vi "modbus slave new.vi"() -> ()   [LabVIEW 2016]
uses:
  <vilib>/NI/Modbus Library/Network Protocol/Network Slave/daemon status.ctl
  <vilib>/NI/Modbus Library/Network Protocol/Network Slave/TCP/Connection.ctl
  <vilib>/NI/Modbus Library/API/Wrapper/Create TCP Slave.vi
  <vilib>/NI/Modbus Library/API/slave/Modbus Slave.lvclass
  <vilib>/NI/Modbus Library/API/Wrapper/API Main.lvlib
  <vilib>/ptbypt/NI_PtbyPt.lvlib
  <vilib>/Utility/config.llb/NI_LVConfig.lvlib
  <vilib>/NI/Modbus Library/Network Protocol/Network Slave/Network Slave.lvclass
  <vilib>/NI/Modbus Library/Network Protocol/Network Slave/TCP/TCP Slave.lvclass
panel:
  out "TCP Connection List":T1[](array[typedef])
  out "TCP Connection Count":u32
  out "Daemon Status":T2
  out "Daemon Error":errorcluster
  out "读取register values 2":u16[](array[numeric])
  out "status":bool
  in  "写入registers to write":u16[](array[numeric])
  out "读取register values":u16[](array[numeric])
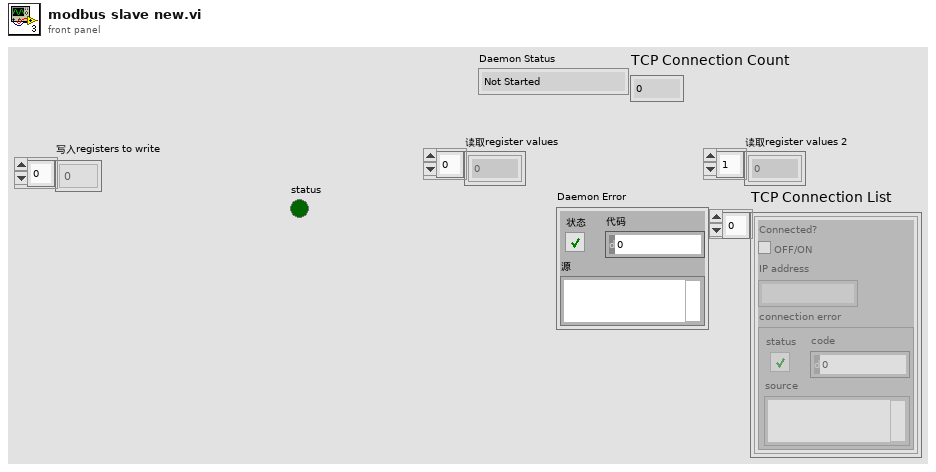
[diagram p1: front panel]
types:
  T1 = typedef "TCP Slave.lvclass/Connection.ctl" = cluster{"Connected?":bool, "IP address":string, "connection error":errorcluster}
  T2 = typedef "Network Slave.lvclass/daemon status.ctl" = enum16{"Not Started", "Running", "Error", "Stopped"}
  T3 = enum16{"启动整机", "停止整机", "标样核查", "加标回收", "平行样测试", "零点核查", "跨度核查", "校零", "校标"}
  T4 = cluster{"status":bool, "代码":u16, "source":string}
  T5 = cluster{"COD浓度（mg/L)":dbl, "水样启动时间":timestamp, "加标回收启动时间":timestamp, "CODMn工作状态":enum16{"空闲", "水样测试", "标样核查", "零点核查", "跨度核查", "空白测试", "平行样测试", "加标回收", "空白校准", "标样校准", "初始化（清洗）"}, "多列列表框":i32}
  T6 = cluster{"系统时间":timestamp, "工作状态":enum16{"空闲", "水样测试", "标样核查", "零点核查", "跨度核查", "空白测试", "平行样测试", "加标回收", "空白校准", "标样校准", "初始化（清洗）"}, "测量模式":enum16{"待机", "连续模式", "周期模式", "定点模式", "受控模式", "手动模式"}, "告警代码":u16, "故障代码":u16, "日志代码":u16, "软件版本":u16, "F0":sgl, "F1":sgl, "F2":sgl, "F3":sgl, "T":sgl, "H":sgl, "id":u16, "flowid":u16, "量程":u16, "总磷控温温度1":sgl, "营养盐控温温度2":sgl, "ADC":sgl}
  T7 = cluster{"系统时间":timestamp, "工作状态":u16, "测量模式":u16, "告警代码":u16, "故障代码":u16, "日志代码":u16, "软件版本":u16, "F0":sgl, "F1":sgl, "F2":sgl, "F3":sgl, "T":sgl, "H":sgl, "id":u16, "flowid":u16, "量程":u16}
  T8 = enum16{"空闲", "水样测试", "标样核查", "零点核查", "跨度核查", "空白测试", "平行样测试", "加标回收", "空白校准", "标样校准", "初始化（清洗）"}
  T9 = typedef "NI_LVConfig.lvlib/Config Data RefNum.ctl" = refnum<k1>
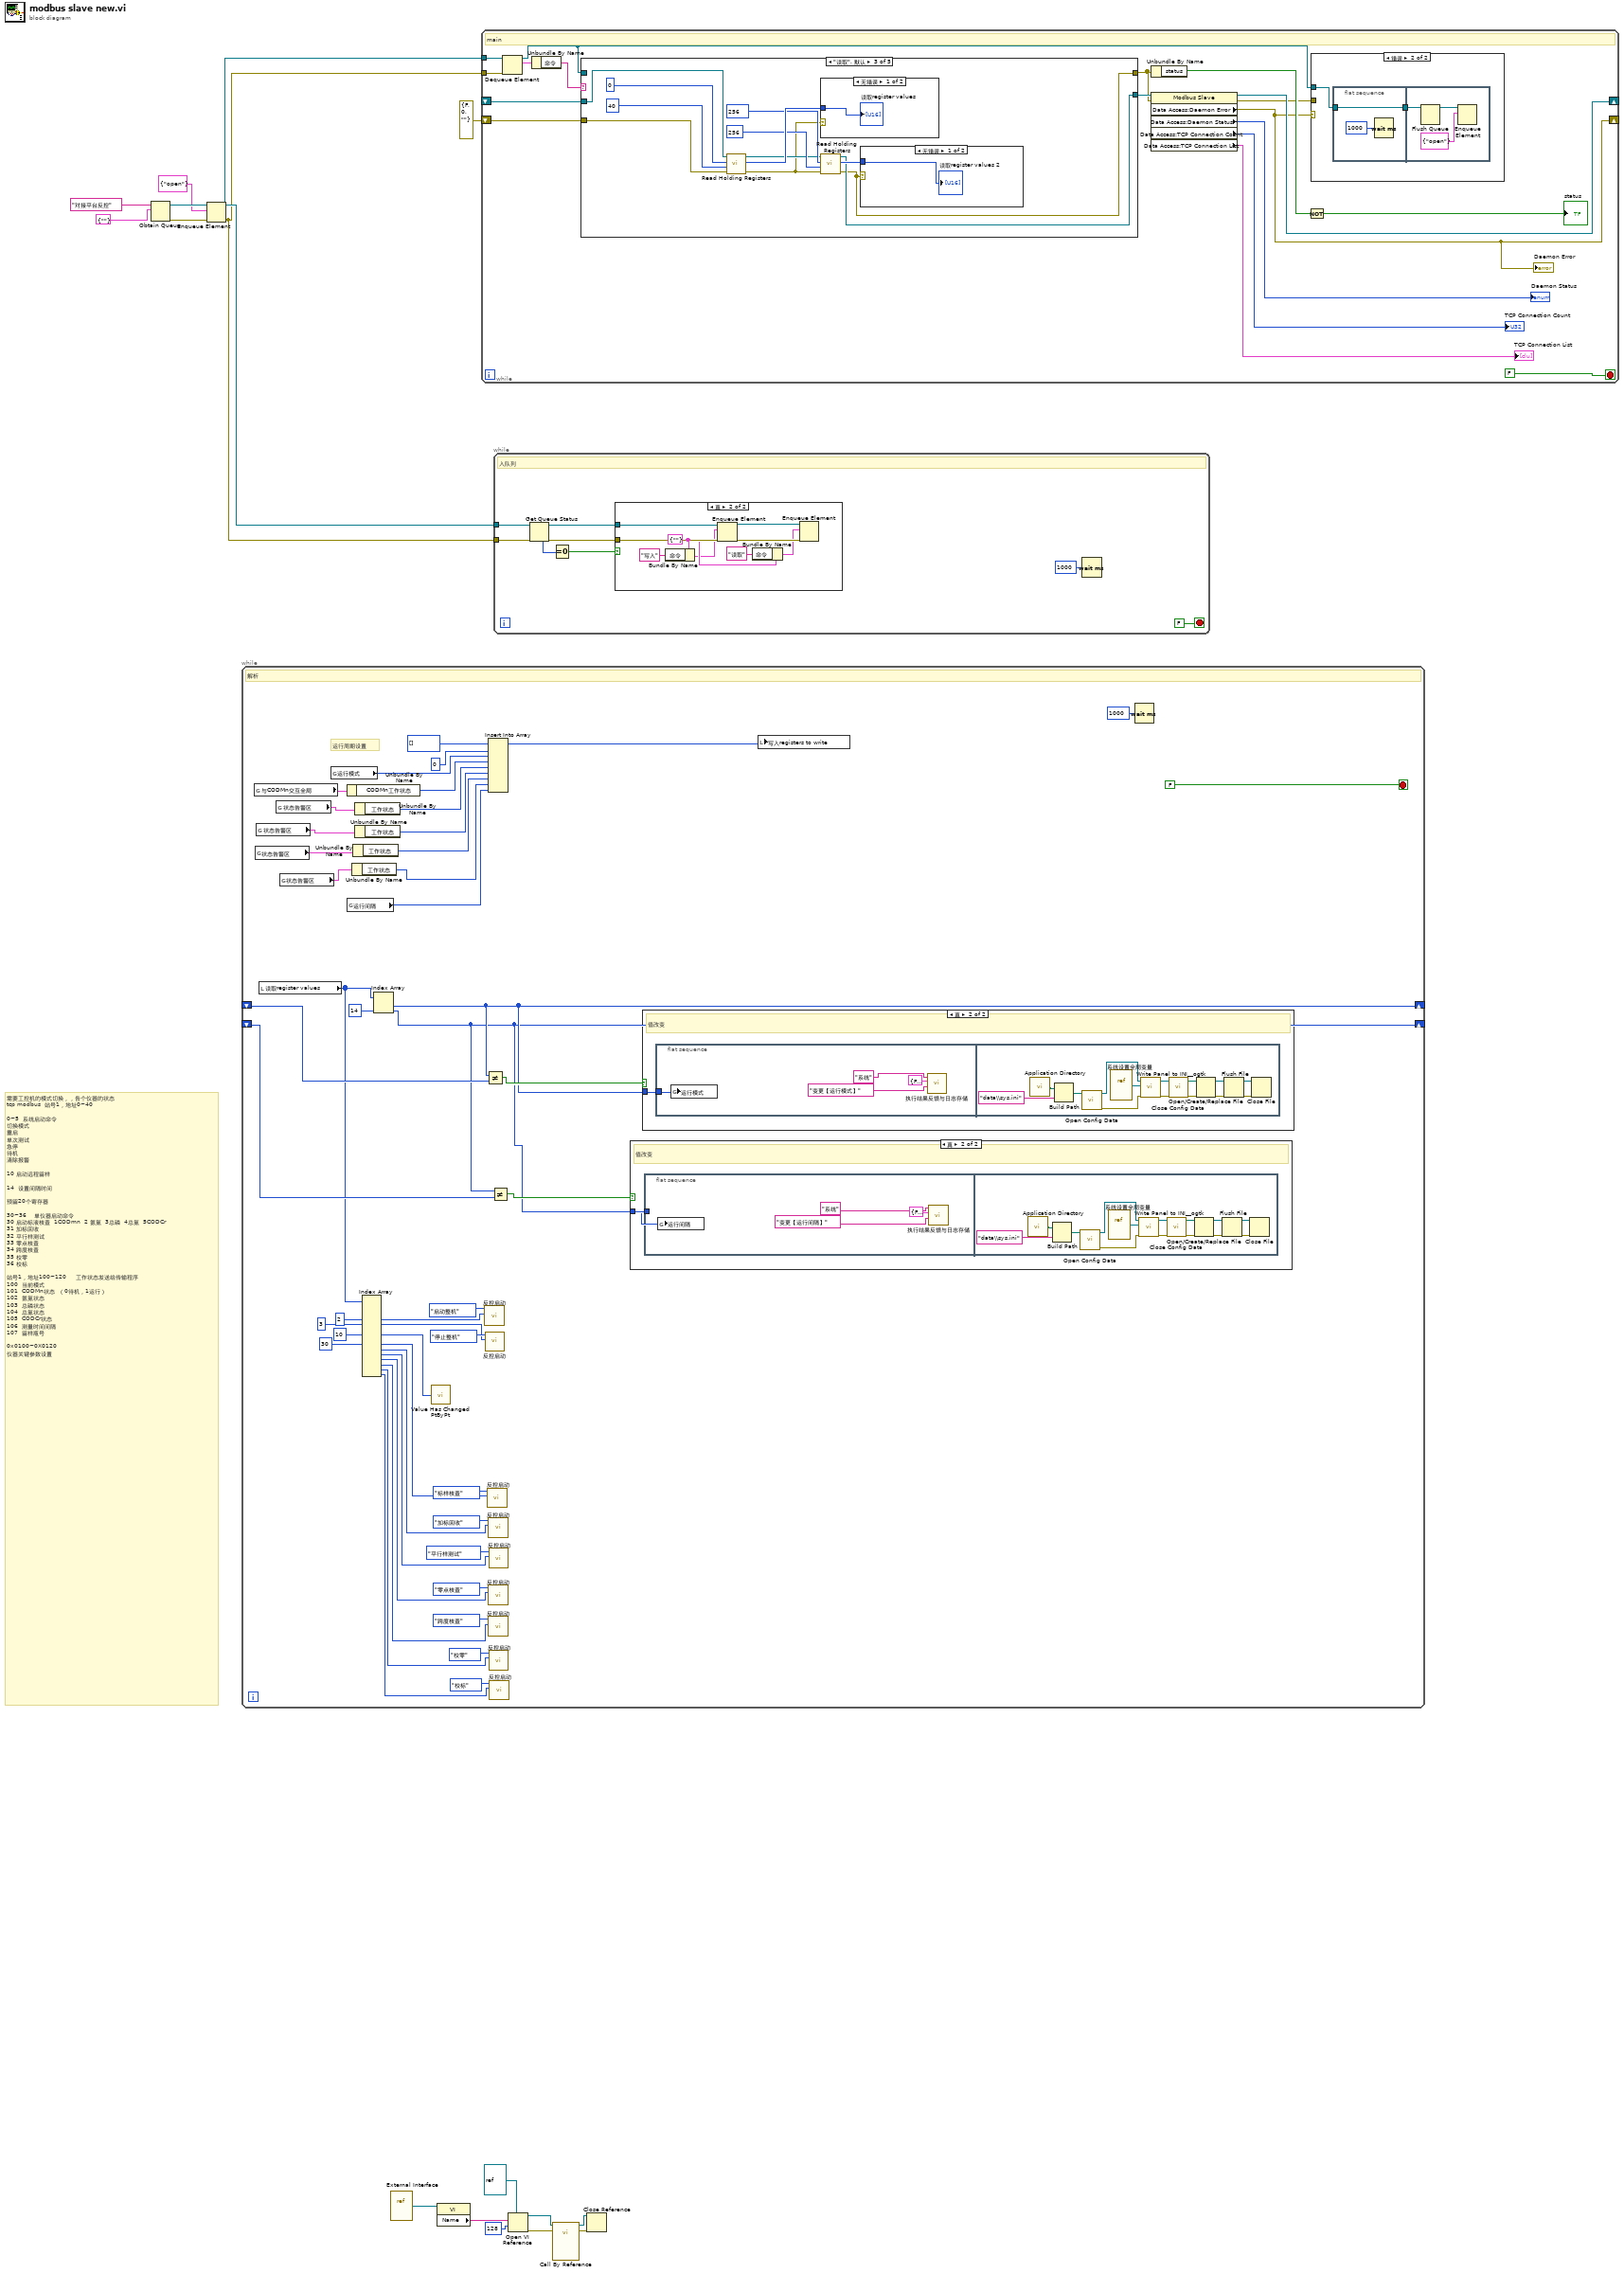
[diagram p0: block diagram]
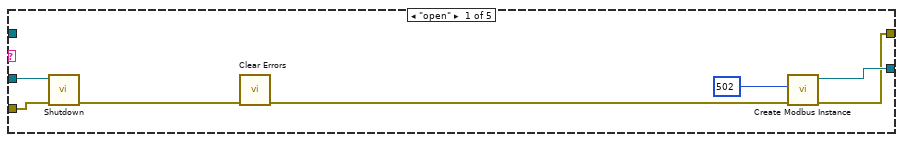
[diagram p6: hidden frame]
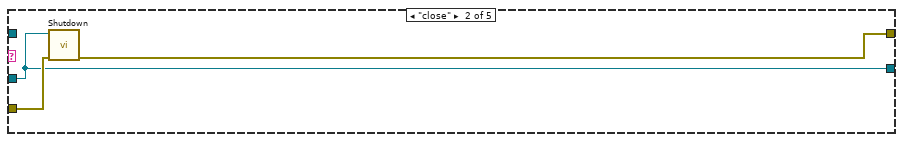
[diagram p7: hidden frame]
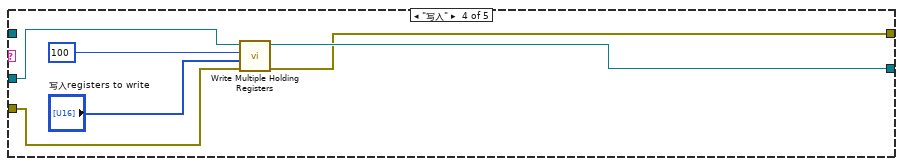
[diagram p10: hidden frame]
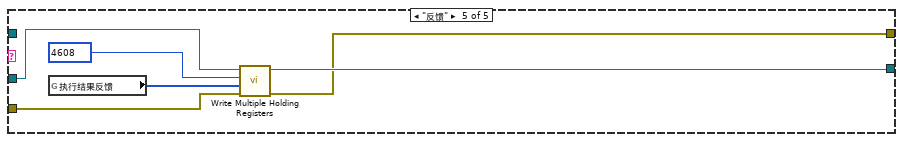
[diagram p11: hidden frame]
diagram:
  # "需要工控机的模式切换，，各个仪器的状态\ntcp modbus  站号1，地址0~40\n\n0~5  系统启动命令\n切换模式\n重启\n单次测试\n急停\n待机\n清除报警\n\n10 启动远程留样\n\n14  设置间隔时间\n\n预留20个寄存器\n\n30~36    单仪器启动命令\n30 启动标液核查  1CODmn  2 氨氮  3总磷  4总氮  5CODCr\n31 加标回收\n32 平行样测试\n33 零点核查\n34 跨度核查\n35 校零\n36 校标\n\n站号1，地址100~120     工作状态发送给传输程序\n100  当前模式\n101  CODMn状态  （0待机，1运行）\n102  氨氮状态\n103  总磷状态\n104  总氮状态\n105  CODCr状态\n106  测量时间间隔\n107  留样瓶号\n\n0x0100~0X0120\n仪器关键参数设置"
  n1 = Obtain Queue(name (unnamed)="对接平台反控" ("名称（未命名）"), element data type=cluster{"命令":string} {"命令"=""}) -> (queue out=w14:refnum<queue>, error out=w13:errorcluster)  [unwired: 3 in, 1 out]
  n2 = Enqueue Element(queue=w14, element=cluster{"命令":string} {"命令"="open"} ("元素"), error in (no error)=w13) -> (queue out=w11:refnum<queue>, error out=w10:errorcluster)  [unwired: 1 in, 1 out]
  n3 = while {
    shift-right: [w51] -> _
    shift-left: _ -> [w53]
    shift-right: [w48] -> _
    shift-left: _ -> [w50]
    stop <- FALSE stop-if-true
    # "运行周期设置"
    # "解析"
    n4 = global read "modbus slave全局.vi" "与CODMn交互全局"() -> (w23:T5)
    n5 = global read "VAR总磷总氮全局变量.vi" "状态告警区"() -> (w17:T6)
    n6 = global read "VAR总磷总氮全局变量.vi" "状态告警区"() -> (w18:T6)
    n7 = local read "读取register values"() -> (w43:u16[])
    n8 = global read "VAR氨氮全局变量.vi" "状态告警区"() -> (w21:T6)
    n9 = global read "CODcr全局变量.vi" "状态告警区"() -> (w20:T7)
    n10 = global read "系统设置全局变量.vi" "运行模式"() -> (w61:enum16{"维护模式", "常规模式", "应急模式", "质控模式"})
    n11 = Unbundle By Name(w23) -> ("CODMn工作状态"=w22:T8)
    n12 = global read "系统设置全局变量.vi" "运行间隔"() -> (w56:i16)
    n13 = Unbundle By Name(w20) -> ("工作状态"=w19:u16)
    n14 = Unbundle By Name(w17) -> ("工作状态"=w57:T8)
    n15 = Unbundle By Name(w21) -> ("工作状态"=w59:T8)
    n16 = Unbundle By Name(w18) -> ("工作状态"=w58:T8)
    n17 = Index Array(array=w43, index #3=2 ("索引"), index #4=3 ("索引"), index #6=10 ("索引"), index #8=30 ("索引")) -> (element #3=w42:u16, element #4=w39:u16, element #6=w38:u16, element #8=w36:u16, element #9=w30:u16, element #10=w29:u16, element #11=w28:u16, element #12=w26:u16, element #13=w25:u16, element #14=w24:u16)  [unwired: 10 in, 4 out]
    n18 = Index Array(array=w43, index #2=14 ("索引")) -> (element #1=w51:u16, element #2=w48:u16)  [unwired: 1 in]
    n19 = call <vilib>:"Value Has Changed PtByPt.vi"("input data point"=w38) -> ()  [unwired: 1 in, 2 out]
    n20 = call "反控启动.vi"("启动参数"=w42, "启动类型"=T3."启动整机") -> ()  [unwired: 10 in]
    n21 = call "反控启动.vi"("启动参数"=w39, "启动类型"=T3."停止整机") -> ()  [unwired: 10 in]
    n22 = Not Equal?(x=w51, y=w53) -> (x != y?=w52:bool)
    n23 = call "反控启动.vi"("启动参数"=w36, "启动类型"=T3."标样核查") -> ()  [unwired: 10 in]
    n24 = Insert Into Array(array=u16[] [] ("values to write"), index=0 ("索引"), new element #1=w61, new element #2=w22, new element #3=w59, new element #4=w58, new element #5=w57, new element #6=w19, new element #7=w56) -> (w55:u16[])
    n25 = call "反控启动.vi"("启动参数"=w30, "启动类型"=T3."加标回收") -> ()  [unwired: 10 in]
    n26 = call "反控启动.vi"("启动参数"=w28, "启动类型"=T3."零点核查") -> ()  [unwired: 10 in]
    n27 = call "反控启动.vi"("启动参数"=w26, "启动类型"=T3."跨度核查") -> ()  [unwired: 10 in]
    n28 = call "反控启动.vi"("启动参数"=w29, "启动类型"=T3."平行样测试") -> ()  [unwired: 10 in]
    n29 = call "反控启动.vi"("启动参数"=w25, "启动类型"=T3."校零") -> ()  [unwired: 10 in]
    n30 = call "反控启动.vi"("启动参数"=w24, "启动类型"=T3."校标") -> ()  [unwired: 10 in]
    n31 = Not Equal?(x=w48, y=w50) -> (x != y?=w49:bool)
    n32 = case shown="真" w49 {
      tunnel: w48 -> [_ w65]
      frame False {
      }
      frame True {
        # "值改变"
        n33 = flat-sequence {
          tunnel: w65 -> [w69]
          frame #0 {
            n34 = global write "系统设置全局变量.vi" "运行间隔"(w69) -> ()
            n35 = call "执行结果反馈与日志存储.vi"("日志信息"="变更【运行间隔】", "error out"=T4 {"status"=FALSE, "代码"=1, "source"=""}, "设备"="系统") -> ()  [unwired: 9 in]
          }
          frame #1 {
            n36 = call <vilib>:"Application Directory.vi"() -> ("Application Directory"=w83:path)
            n37 = Build Path(base path=w83, name or relative path="data\\sys.ini" ("名称或相对路径")) -> (appended path=w81:path)
            n38 = call <vilib>:"Open Config Data.vi"("configuration file path"=w81) -> ("error out"=w77:errorcluster, "refnum"=w80:T9)  [unwired: 8 in, 1 out]
            n39 = vi-ref "系统设置全局变量.vi"() -> (w79:refnum<vi>)
            n40 = call <userlib>:"Write Panel to INI__ogtk.vi"("error in (no error)"=w77, "VI ref"=w79, "refnum"=w80) -> ("error out"=w76:errorcluster, "refnum out"=w78:T9)  [unwired: 7 in]
            n41 = call <vilib>:"Close Config Data.vi"("error in (no error)"=w76, "refnum"=w78) -> ("error out"=w71:errorcluster, "file path"=w70:path)  [unwired: 8 in]
            n42 = Open/Create/Replace File(file path (use dialog)=w70, error in=w71) -> (refnum out=w74:refnum<file>, error out=w75:errorcluster)  [unwired: 4 in, 1 out]
            n43 = Flush File(refnum=w74, error in=w75) -> (refnum out=w73:refnum<file>, error out=w72:errorcluster)
            n44 = Close File(refnum=w73, error in=w72) -> ()  [unwired: 2 out]
          }
        }
      }
    }
    n45 = case shown="真" w52 {
      tunnel: w51 -> [_ w84]
      frame False {
      }
      frame True {
        # "值改变"
        n46 = flat-sequence {
          tunnel: w84 -> [w88]
          frame #0 {
            n47 = global write "系统设置全局变量.vi" "运行模式"(w88) -> ()
            n48 = call "执行结果反馈与日志存储.vi"("日志信息"="变更【运行模式】", "error out"=T4 {"status"=FALSE, "代码"=1, "source"=""}, "设备"="系统") -> ()  [unwired: 9 in]
          }
          frame #1 {
            n49 = call <vilib>:"Application Directory.vi"() -> ("Application Directory"=w102:path)
            n50 = Build Path(base path=w102, name or relative path="data\\sys.ini" ("名称或相对路径")) -> (appended path=w100:path)
            n51 = call <vilib>:"Open Config Data.vi"("configuration file path"=w100) -> ("error out"=w96:errorcluster, "refnum"=w99:T9)  [unwired: 8 in, 1 out]
            n52 = vi-ref "系统设置全局变量.vi"() -> (w98:refnum<vi>)
            n53 = call <userlib>:"Write Panel to INI__ogtk.vi"("error in (no error)"=w96, "VI ref"=w98, "refnum"=w99) -> ("error out"=w95:errorcluster, "refnum out"=w97:T9)  [unwired: 7 in]
            n54 = call <vilib>:"Close Config Data.vi"("error in (no error)"=w95, "refnum"=w97) -> ("error out"=w90:errorcluster, "file path"=w89:path)  [unwired: 8 in]
            n55 = Open/Create/Replace File(file path (use dialog)=w89, error in=w90) -> (refnum out=w93:refnum<file>, error out=w94:errorcluster)  [unwired: 4 in, 1 out]
            n56 = Flush File(refnum=w93, error in=w94) -> (refnum out=w92:refnum<file>, error out=w91:errorcluster)
            n57 = Close File(refnum=w92, error in=w91) -> ()  [unwired: 2 out]
          }
        }
      }
    }
    n58 = local write "写入registers to write"(w55) -> ()
    n59 = Wait (ms)(milliseconds to wait=u32 1000 ("等待时间（毫秒）")) -> ()  [unwired: 1 out]
  }
  n60 = vi-ref "External Interface.vi"() -> (w9:refnum<vi>)
  n61 = property class="VI"(reference=w9) -> ("Name"=w8:string)  [unwired: 1 in, 2 out]
  n62 = while {
    tunnel: w11 -> [w120]
    tunnel: w10 -> [w119]
    shift-right: [w109] -> _
    shift-left: _ -> [w107]
    shift-right: [w103] -> _
    shift-left: errorcluster {"status"=FALSE, "code"=0, "source"=""} ("error out") -> [w108]
    stop <- FALSE stop-if-true
    # "main"
    n63 = Dequeue Element(queue=w120, error in (no error)=w119) -> (queue out=w105:refnum<queue>, element=w118:cluster{"命令":string})  [unwired: 1 in, 2 out]
    n64 = Unbundle By Name(w118) -> ("命令"=w117:string)
    n65 = case shown="\"读取\", 默认" w117 {
      tunnel: [w129 w135 w139 w153 w160] -> w113
      tunnel: [w128 w136 w138 w152 w159] -> w106
      tunnel: w107 -> [w133 w135 w149 w157 w162]
      tunnel: w108 -> [w132 w137 w148 w156 w161]
      tunnel: w105 -> [_ _ _ _ _]
      frame "open" {
        n66 = call-dynamic "Shutdown.vi"("error in"=w132, "Modbus slave in"=w133) -> ("error out"=w131:errorcluster)  [unwired: 9 in]
        n67 = call <vilib>:"Clear Errors.vi"("error in (no error)"=w131) -> ("error out"=w130:errorcluster)  [unwired: 5 in, 1 out]
        n68 = call-poly <vilib>:"Create Modbus Instance.vi"("error in"=w130, "port (502)"=u16 502) -> ("error out"=w128:errorcluster, "TCP slave instance"=w129:refnum<class "Modbus Slave.lvclass">)  [unwired: 8 in]
      }
      frame "close" {
        n69 = call-dynamic "Shutdown.vi"("error in"=w137, "Modbus slave in"=w135) -> ("error out"=w136:errorcluster)  [unwired: 9 in]
      }
      frame "读取", Default {
        n70 = call-dynamic "Read Holding Registers.vi"("error in"=w148, "number of inputs"=u16 40, "starting address"=u16 0, "Modbus slave in"=w149) -> ("error out"=w140:errorcluster, "register values"=w145:u16[], "Modbus slave out"=w141:refnum<class "Modbus Slave.lvclass">)  [unwired: 5 in]
        n71 = case shown="无错误" w140 {
          tunnel: w145 -> [w151 _]
          frame No Error {
            "读取register values" <- w151
          }
          frame Error {
          }
        }
        n72 = call-dynamic "Read Holding Registers.vi"("error in"=w140, "number of inputs"=u16 256, "starting address"=u16 256, "Modbus slave in"=w141) -> ("error out"=w138:errorcluster, "register values"=w144:u16[], "Modbus slave out"=w139:refnum<class "Modbus Slave.lvclass">)  [unwired: 5 in]
        n73 = case shown="无错误" w138 {
          tunnel: w144 -> [w150 _]
          frame No Error {
            "读取register values 2" <- w150
          }
          frame Error {
          }
        }
      }
      frame "写入" {
        n74 = call-dynamic "Write Multiple Holding Registers.vi"("error in"=w156, "registers to write"="写入registers to write", "starting address"=u16 100, "Modbus slave in"=w157) -> ("error out"=w152:errorcluster, "Modbus slave out"=w153:refnum<class "Modbus Slave.lvclass">)  [unwired: 6 in]
      }
      frame "反馈" {
        n75 = global read "modbus slave全局.vi" "执行结果反馈"() -> (w158:u16[])
        n76 = call-dynamic "Write Multiple Holding Registers.vi"("error in"=w161, "registers to write"=w158, "starting address"=u16 4608, "Modbus slave in"=w162) -> ("error out"=w159:errorcluster, "Modbus slave out"=w160:refnum<class "Modbus Slave.lvclass">)  [unwired: 6 in]
      }
    }
    n77 = Unbundle By Name(w106) -> ("status"=w115:bool)
    n78 = property class="Modbus Slave"(reference=w113, error in=w106) -> (reference out=w109:refnum<class "Modbus Slave.lvclass">, error out=w104:errorcluster, "Data Access:Daemon Error"=w103:errorcluster, "Data Access:Daemon Status"=→"Daemon Status":T2, "Data Access:TCP Connection Count"=→"TCP Connection Count":u32, "Data Access:TCP Connection List"=→"TCP Connection List":T1[])
    "Daemon Error" <- w103
    n79 = Not(x=w115) -> (.not. x?=→"status":bool)
    n80 = case shown="错误" w103 {
      tunnel: w105 -> [_ w122]
      tunnel: w104 -> [_ _]
      frame No Error {
      }
      frame Error {
        n81 = flat-sequence {
          tunnel: w122 -> [w124]
          tunnel: [w124] -> w121
          tunnel: w121 -> [w127]
          frame #0 {
            n82 = Wait (ms)(milliseconds to wait=u32 1000 ("等待时间（毫秒）")) -> ()  [unwired: 1 out]
          }
          frame #1 {
            n83 = Flush Queue(queue=w127) -> (queue out=w125:refnum<queue>)  [unwired: 1 in, 2 out]
            n84 = Enqueue Element(queue=w125, element=cluster{"命令":string} {"命令"="open"} ("元素")) -> ()  [unwired: 2 in, 3 out]
          }
        }
      }
    }
  }
  n85 = while {
    tunnel: w11 -> [w171]
    tunnel: w10 -> [w169]
    stop <- FALSE stop-if-true
    # "入队列"
    n86 = Get Queue Status(queue=w171, error in (no error)=w169) -> (queue out=w170:refnum<queue>, error out=w168:errorcluster, # elements in queue=w167:i32)  [unwired: 1 in, 5 out]
    n87 = Equal To 0?(x=w167) -> (x = 0?=w166:bool)
    n88 = case shown="真" w166 {
      tunnel: w170 -> [_ w180]
      tunnel: w168 -> [_ w179]
      frame False {
      }
      frame True {
        w175 = cluster{"命令":string} {"命令"=""} ("元素")
        n89 = Bundle By Name(cluster=w175, "命令"="写入") -> (w174:cluster{"命令":string})
        n90 = Enqueue Element(queue=w180, element=w174, error in (no error)=w179) -> (queue out=w178:refnum<queue>, error out=w177:errorcluster)  [unwired: 1 in, 1 out]
        n91 = Bundle By Name(cluster=w175, "命令"="读取") -> (w172:cluster{"命令":string})
        n92 = Enqueue Element(queue=w178, element=w172, error in (no error)=w177) -> ()  [unwired: 1 in, 3 out]
      }
    }
    n93 = Wait (ms)(milliseconds to wait=u32 1000 ("等待时间（毫秒）")) -> ()  [unwired: 1 out]
  }
  n94 = Open VI Reference(type specifier VI Refnum (for type only)=refnum<vi> refnum, vi path=w8, options=128 ("选项")) -> (vi reference=w6:refnum<vi>, error out=w4:errorcluster)  [unwired: 3 in]
  n95 = call-by-ref "?"(reference=w6, error in=w4) -> (reference out=w2:refnum<vi>, error out=w3:errorcluster)  [unwired: 12 in]
  n96 = Close Reference(reference=w2, error in (no error)=w3) -> ()  [unwired: 1 out]
